vi "Polar To Rectangular.vi"(2 "phase":dbl format="%0.2f", 3 "magnitude":dbl format="%0.2f") -> (0 "y":dbl format="%0.2f", 1 "x":dbl format="%0.2f")   [LabVIEW 2018, in "NI_AALPro.lvlib"]
doc: "Converts the set of polar coordinates represented by the input values, magnitude and phase, to rectangular coordinates."
uses:
  NI_AALPro.lvlib
panel:
  # "Polar To Rectangular"
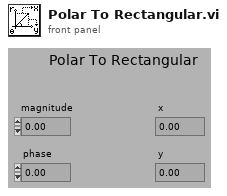
[diagram p1: front panel]
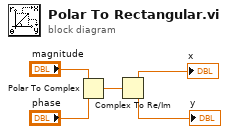
[diagram p0: block diagram]
diagram:
  n1 = Polar To Complex(1:"phase", 2:"magnitude") -> (0:w5:cdb)
  n2 = Complex To Re/Im(x + iy=w5) -> (x=→"x":dbl, y=→"y":dbl)
